vi "UHR-Fleezers Control (host) -Leonardo 04-2018 V3.vi"(0 "Tab Control":T5(tab)=enum."Trap Control (RF)") -> ()   [LabVIEW 2013] (continued)
                n951 = Unbundle By Name(w1533) -> ("Pump 2"=w1539:T33)
                n952 = call "Set pump parameters.vi"("Pump write delay (ms)"=w1534, "Volume (uL)"="Flush Center Ch Volume (uL)", "Rate (uL/h)"=w1530, "Units"=3.0, "Pump #"=2.0, "Pump Parameters In"=w1539, "VISA resource name"=w1538) -> ("Pump Parameters Out"=w1532:T33)  [unwired: 3 in]
                n953 = Bundle By Name(cluster=w1533, "Pump 2"=w1532) -> (w1531:T6)
                n954 = local write "All Pump Parameters"(w1531) -> ()
                n955 = Add(x="Flush Center Ch Volume (uL)", y="Total Volume\nFlushed (uL)") -> (x+y=w1527:dbl)
                n956 = local write "Total Volume\nFlushed (uL)"(w1527) -> ()
              }
              frame #1 {
                n957 = Wait (ms)(milliseconds to wait=w1540) -> ()  [unwired: 1 out]
              }
              frame #2 {
                n958 = call "Write to pump.vi"("string"="start", "VISA resource name"=w1541) -> ()  [unwired: 1 out]
              }
            }
            n959 = local read "Chemyx Syringe Pump Serial Port"() -> (w1524:refnum<visa-resource-name>)
          }
          frame Enabled {
            n960 = call "hamilton_controller.vi"("Open?"=w1543, "valve"=enum16{"A", "B", "C", "D", "ALL"}."B", "action"=T21."MOVE VALVE") -> ()  [unwired: 8 in, 1 out]
          }
        }
      }
      event "Inject Bottom": Value Change {
        n961 = event-data() -> ()  [unwired: 7 out]
        n962 = call "hamilton_controller.vi"("Open?"="Inject Bottom", "valve"=enum16{"A", "B", "C", "D", "ALL"}."C", "action"=T21."MOVE VALVE") -> ()  [unwired: 8 in, 1 out]
      }
      event "Shunt:": Value Change {
        n963 = event-data() -> ()  [unwired: 7 out]
        n964 = call "hamilton_controller.vi"("Open?"="Shunt:", "valve"=enum16{"A", "B", "C", "D", "ALL"}."D", "action"=T21."MOVE VALVE") -> ()  [unwired: 8 in, 1 out]
      }
      event "Flip Green Filter": Value Change {
        n965 = event-data() -> ()  [unwired: 7 out]
        n966 = local write "Flip Green Filter"("Flip Green Filter") -> ()
        n967 = flat-sequence {
          tunnel: w1559 -> [w1564]
          tunnel: w1558 -> [w1563]
          tunnel: [w1561] -> w1556
          tunnel: [w1560] -> w1555
          tunnel: [w1566] -> w1554
          tunnel: w1556 -> [w1566]
          tunnel: [w1565] -> w1553
          tunnel: w1555 -> [w1565]
          tunnel: w1554 -> [w1570]
          tunnel: w1553 -> [w1569]
          tunnel: [w1568] -> w1557
          frame #0 {
            n968 = xnode "Read/Write Control"("FPGA VI Reference In"=w1564, "error in"=w1563, "Green Filter Flipper"=TRUE) -> ("FPGA VI Reference Out"=w1561:T20, "error out"=w1560:errorcluster)
          }
          frame #1 {
            n969 = Wait (ms)(milliseconds to wait=u32 100) -> ()  [unwired: 1 out]
          }
          frame #2 {
            n970 = xnode "Read/Write Control"("FPGA VI Reference In"=w1570, "error in"=w1569, "Green Filter Flipper"=FALSE) -> ("error out"=w1568:errorcluster)  [unwired: 1 out]
          }
        }
      }
      event "Pump 1 contents", "Pump 3 contents": Value Change {
        n971 = event-data() -> ()  [unwired: 7 out]
        n972 = local read "Pump 1 contents"() -> (→"Pump 1 cont disp":string)
        n973 = local read "Pump 3 contents"() -> (→"Pump 3 cont disp":string)
      }
      event "Reset Trap Pos. FB": Value Change {
        n974 = event-data() -> ()  [unwired: 7 out]
        n975 = xnode "Read/Write Control"("FPGA VI Reference In"=w1576, "error in"=w1575, "Trap Pos. FB Reset"="Reset Trap Pos. FB") -> ()  [unwired: 2 out]
      }
      event "Trap Pos. FB ON": Value Change {
        n976 = event-data() -> ()  [unwired: 7 out]
        n977 = xnode "Read/Write Control"("FPGA VI Reference In"=w1591, "error in"=w1590) -> ("FPGA VI Reference Out"=w1588:T20, "BD1 Frequency Out 1"=w1585:u64)  [unwired: 1 out]
        n978 = To Double Precision Float(number=w1585) -> (double precision float=w1584:dbl)
        n979 = Multiply(x=49125000.0, y=6.0) -> (x*y=w1583:dbl)
        n980 = Multiply(x=w1584, y=w1583) -> (x*y=w1581:dbl)
        n981 = Scale By Power Of 2(n=-48, x=w1581) -> (x*2^n=w1580:dbl)
        n982 = Divide(x=w1580, y=1000000.0) -> (x/y=w1577:dbl)
        n983 = flat-sequence {
          tunnel: [w1594] -> w1589
          tunnel: w1588 -> [w1595]
          tunnel: w1585 -> [w1593]
          tunnel: "Trap Pos. FB ON" -> [w1592]
          tunnel: "Trap Pos. FB ON" -> [w1601]
          tunnel: w1589 -> [w1600]
          tunnel: "Trap Pos. FB ON" -> [w1603]
          tunnel: w1577 -> [w1602]
          frame #0 {
            n984 = case shown="False" w1592 {
              tunnel: w1595 -> [w1598 w1599]
              tunnel: [w1597 w1599] -> w1594
              tunnel: w1593 -> [w1596 _]
              frame False {
                n985 = xnode "Read/Write Control"("FPGA VI Reference In"=w1598, "BD 1 Frequency 1"=w1596) -> ("FPGA VI Reference Out"=w1597:T20)  [unwired: 1 in, 1 out]
              }
              frame True {
              }
            }
          }
          frame #1 {
            n986 = xnode "Read/Write Control"("FPGA VI Reference In"=w1600, "Force feedback"=w1601) -> ()  [unwired: 1 in, 2 out]
          }
          frame #2 {
            n987 = case shown="False" w1603 {
              tunnel: w1602 -> [w1605 _]
              frame False {
                n988 = Subtract(x=90.0, y=w1605) -> (x-y=w1604:dbl)
                n989 = property on="Trap Delta (MHz)" class="DigNum (strict)"("Val(Sgnl)"=w1604) -> ()  [unwired: 2 in, 2 out]
              }
              frame True {
              }
            }
          }
        }
      }
      event "Diff. FB.", "Trap Pos. FB Gains", "Trap Pos. FB Mult Factor", "Trap Pos. FB Offset Factor", "Trap Pos FB Negate Action", "Trap Pos FB Monitor\nT1 or T2", "Negate Diff?": Value Change {
        n990 = event-data() -> ()  [unwired: 7 out]
        n991 = xnode "Read/Write Control"("FPGA VI Reference In"=w1617, "error in"=w1616, "Trap pos. FB Range"="Trap Pos. FB Range", "Trap Pos. FB Gains"="Trap Pos. FB Gains", "Trap Pos. FB Mult Factor"="Trap Pos. FB Mult Factor", "Trap Pos. FB Offset Factor"="Trap Pos. FB Offset Factor", "Trap Pos FB Negate Action"="Trap Pos FB Negate Action", "Trap Pos FB Monitor T1 or T2"="Trap Pos FB Monitor\nT1 or T2", "AI1 X Scale"="Trap Pos. AI1 X Pre-scale", "Negate Diff?"="Negate Diff?", "Diff FB Measurement?"="Diff. FB.") -> ()  [unwired: 2 out]
      }
      event "Trap Pos FB SP": Value Change {
        n992 = event-data() -> ()  [unwired: 7 out]
        n993 = xnode "Read/Write Control"("FPGA VI Reference In"=w1620, "error in"=w1619, "Trap Pos. FB SP"="Trap Pos FB SP") -> ()  [unwired: 2 out]
      }
      event "Simulate stepping": Value Change {
        n994 = event-data() -> ()  [unwired: 7 out]
        n995 = flat-sequence {
          tunnel: w1622 -> [w1625]
          tunnel: [w1624] -> _
          tunnel: w1621 -> [w1623]
          frame #0 {
            n996 = while {
              tunnel: w1625 -> [w1653]
              tunnel: [w1652] -> w1624 mode=indexing
              tunnel: w1623 -> [w1651]
              i -> [w1637]
              stop <- w1634 stop-if-true
              w1627 = 1000.0
              n997 = Divide(x="Backtrack probability", y=100) -> (x/y=w1661:dbl)
              n998 = Random Number (0-1)() -> (number: 0 to 1=w1662:dbl)
              n999 = Greater?(x=w1662, y=w1661) -> (0:w1660:bool)
              n1000 = Select(t=1, s=w1660, f=-1) -> (s? t:f=w1657:i32)
              n1001 = local read "BD 1 Frequency 2 (MHz)"() -> (w1632:dbl)
              n1002 = Multiply(x=w1657, y="Step size (nm)") -> (x*y=w1655:dbl)
              "Step taken" <- w1655
              n1003 = Divide(x=w1655, y=168.33) -> (x/y=w1630:dbl)
              n1004 = local read "BD 1 Frequency 1 (MHz)"() -> (w1631:dbl)
              n1005 = local read "X RF Frequency Limits (MHz)"() -> (w1650:T16)
              n1006 = local read "Y RF Frequency Limits (MHz)"() -> (w1649:T16)
              n1007 = Subtract(x=w1631, y=w1630) -> (x-y=w1629:dbl)
              n1008 = local write "BD 1 Frequency 1 (MHz)"(w1629) -> ()
              n1009 = local read "BD 2 Frequency 1 (MHz)"() -> (w1647:dbl)
              n1010 = local read "BD 2 Frequency 2 (MHz)"() -> (w1648:dbl)
              n1011 = call "set RF board frequency - interlace.vi"("Board 2 Frequency Limits"=w1649, "Board 1 Frequency Limits"=w1650, "error in"=w1653, "FPGA VI Reference In"=w1651, "Board 2 Frequency 2 (MHz)"=w1648, "Board 2 Frequency 1 (MHz)"=w1647, "Board 1 Frequency 2 (MHz)"=w1632, "Board 1 Frequency 1  (MHz)"=w1629) -> ("error out"=w1652:errorcluster)  [unwired: 2 in, 1 out]
              n1012 = Subtract(x=w1632, y=w1629) -> (x-y=w1646:dbl)
              n1013 = Subtract(x=w1648, y=w1647) -> (x-y=w1645:dbl)
              n1014 = Square(x=w1645) -> (x^2=w1643:dbl)
              n1015 = Square(x=w1646) -> (x^2=w1644:dbl)
              n1016 = Add(x=w1644, y=w1643) -> (x+y=w1642:dbl)
              n1017 = Square Root(x=w1642) -> (sqrt(x)=w1633:dbl)
              n1018 = local write "Trap Delta (MHz)"(w1633) -> ()
              n1019 = property on="Initial delta (MHz)" class="DigNum (strict)"("Val(Sgnl)"=w1633) -> ()  [unwired: 2 in, 2 out]
              n1020 = Multiply(x="Mean dwell time (s)", y=w1627) -> (x*y=w1639:dbl)
              n1021 = case shown="\"Gamma2\"" "Distribution" {
                tunnel: w1639 -> [w1666 w1670 w1673]
                tunnel: [w1666 w1667 w1674] -> w1628
                frame "uniform", Default {
                }
                frame "Exponential" {
                  n1022 = call-poly <vilib>:"Continuous Random.vi"("b"=w1670, "samples"=1) -> ("exp random data"=w1668:dbl[])  [unwired: 8 in, 1 out]
                  n1023 = Index Array(array=w1668) -> (element=w1667:dbl)  [unwired: 1 in]
                }
                frame "Gamma2" {
                  w1671 = 2.0
                  # "Note: the shape and scale\nparameters of the gamma\nare inverted because LabView..."
                  n1024 = Divide(x=w1673, y=w1671) -> (x/y=w1672:dbl)
                  n1025 = call-poly <vilib>:"Continuous Random.vi"("c"=w1672, "b"=w1671, "samples"=1) -> ("gamma random numbers"=w1675:dbl[])  [unwired: 7 in, 1 out]
                  n1026 = Index Array(array=w1675) -> (element=w1674:dbl)  [unwired: 1 in]
                }
              }
              n1027 = Divide(x=w1628, y=w1627) -> (x/y=→"Step duration":dbl)
              n1028 = To Unsigned Long Integer(number=w1628) -> (unsigned 32bit integer=w1640:u32)
              n1029 = Add(x=w1637, y=1) -> (x+y=w1636:i32)
              n1030 = Wait (ms)(milliseconds to wait=w1640) -> ()  [unwired: 1 out]
              n1031 = Equal?(x=w1636, y="Number of steps") -> (x = y?=w1634:bool)
            }
          }
          frame #1 {
            n1032 = local write "Simulate stepping"(FALSE) -> ()
          }
        }
      }
      event "Set SP to Reading": Value Change {
        n1033 = event-data() -> ()  [unwired: 7 out]
        n1034 = local read "Trap Pos FB Monitor\nT1 or T2"() -> (w1685:bool)
        n1035 = local read "Trap X AI1 (DMA)"() -> (w1688:T13)
        n1036 = local read "Trap X (AI1)"() -> (w1691:T1)
        n1037 = Unbundle By Name(w1691) -> ("Trap 1"=w1690:fxp<+/-,16,1>, "Trap 2"=w1689:fxp<+/-,16,1>)
        n1038 = Unbundle By Name(w1688) -> ("Set 1"=w1687:fxp<+/-,16,1>, "Set 2"=w1686:fxp<+/-,16,1>)
        n1039 = Select(t=w1690, s=w1685, f=w1689) -> (s? t:f=w1684:fxp<+/-,16,1>)
        n1040 = Select(t=w1687, s=w1685, f=w1686) -> (s? t:f=w1683:fxp<+/-,16,1>)
        n1041 = Not(x="Set SP Using...") -> (.not. x?=w1678:bool)
        n1042 = Select(t=w1684, s=w1678, f=w1683) -> (s? t:f=w1679:fxp<+/-,16,1>)
        n1043 = xnode "Read/Write Control"("FPGA VI Reference In"=w1681, "error in"=w1680, "Trap Pos. FB SP"=w1679) -> ()  [unwired: 2 out]
        n1044 = local write "Trap Pos FB SP"(w1679) -> ()
      }
      event "Trap Pos. FB Out Scale 2^n": Value Change {
        n1045 = event-data() -> ()  [unwired: 7 out]
        n1046 = Scale By Power Of 2(n="Trap Pos. FB Out Scale 2^n", x=ext 1.0) -> (x*2^n=w1693:ext)
        n1047 = property on="Trap Pos. FB Mult Factor" class="DigNum (strict)"("Val(Sgnl)"=w1693) -> ()  [unwired: 2 in, 2 out]
      }
      event "Trap Pos FB Int Count": Value Change {
        n1048 = event-data() -> ()  [unwired: 7 out]
        n1049 = xnode "Read/Write Control"("FPGA VI Reference In"=w1698, "error in"=w1697, "Trap Pos FB Int Count"="Trap Pos FB Int Count") -> ()  [unwired: 2 out]
      }
      event "Target Force (pN)", "Setpoint offset\nCorrection values", "Raster target force (pN)": Value Change {
        w1706 = 2.0
        n1050 = event-data() -> ()  [unwired: 7 out]
        n1051 = local read "B factor"() -> (w1737:dbl)
        n1052 = To Fixed-Point(number=w1737) -> (fixed-point=w1736:fxp<+/-,16,16>)  [unwired: 1 in]
        n1053 = xnode "Read/Write Control"("FPGA VI Reference In"=w1700, "B factor"=w1736) -> ("BD1 Frequency Out 1"=w1727:u64)  [unwired: 1 in, 2 out]
        n1054 = local read "BD 1 Frequency 2 (MHz)"() -> (w1726:dbl)
        n1055 = local read "Target Force (pN)"() -> (w1712:dbl)
        n1056 = To Double Precision Float(number=w1727) -> (double precision float=w1733:dbl)
        n1057 = Multiply(x=49125000.0, y=6.0) -> (x*y=w1732:dbl)
        n1058 = Multiply(x=w1733, y=w1732) -> (x*y=w1730:dbl)
        n1059 = Scale By Power Of 2(n=-48, x=w1730) -> (x*2^n=w1729:dbl)
        n1060 = Divide(x=w1729, y=1000000.0) -> (x/y=w1725:dbl)
        n1061 = Subtract(x=w1726, y=w1725) -> (x-y=w1724:dbl)
        n1062 = local read "T1 kappa_x (pN/nm)"() -> (w1713:dbl)
        n1063 = local read "T1 alpha_x (nm/V)"() -> (w1714:dbl)
        n1064 = local read "Negate offset difference"() -> (w1715:bool)
        n1065 = local read "Offset file step size"() -> (w1723:dbl)
        n1066 = Multiply(x="Raster target force (pN)", y=w1706) -> (x*y=w1705:dbl)
        n1067 = Multiply(x=w1712, y=w1706) -> (x*y=w1711:dbl)
        n1068 = local read "Setpoint offset\nCorrection values"() -> (w1720:dbl[])
        n1069 = Divide(x=w1724, y=w1723) -> (x/y=w1722:dbl)
        n1070 = Select(t=-1, s=w1715, f=1) -> (s? t:f=w1716:i32)
        n1071 = To Long Integer(number=w1722) -> (32bit integer=w1721:i32)
        n1072 = Multiply(x=w1714, y=w1713) -> (x*y=w1704:dbl)
        n1073 = Divide(x=w1711, y=w1704) -> (x/y=w1710:dbl)
        n1074 = Index Array(array=w1720, index=w1721) -> (element=w1719:dbl)
        n1075 = Divide(x=w1705, y=w1704) -> (x/y=w1703:dbl)
        n1076 = Multiply(x=w1716, y=w1719) -> (x*y=w1702:dbl)
        n1077 = Add(x=w1710, y=w1702) -> (x+y=w1709:dbl)
        n1078 = Add(x=w1703, y=w1702) -> (x+y=w1701:dbl)
        n1079 = To Fixed-Point(number=w1701) -> (fixed-point=w1699:fxp<+/-,16,1>)  [unwired: 1 in]
        n1080 = To Fixed-Point(number=w1709) -> (fixed-point=w1708:fxp<+/-,16,1>)  [unwired: 1 in]
        n1081 = property on="Trap Pos FB SP" class="DigNum (strict)"("Val(Sgnl)"=w1708) -> ()  [unwired: 2 in, 2 out]
        n1082 = xnode "Read/Write Control"("FPGA VI Reference In"=w1700, "Raster setpoint"=w1699) -> ()  [unwired: 1 in, 2 out]
      }
      event "Read setpoint correction\nfile": Value Change {
        n1083 = event-data() -> ()  [unwired: 7 out]
        n1084 = local write "Read setpoint correction\nfile"(FALSE) -> ()
        n1085 = Open/Create/Replace File(file path (use dialog)="Setpoint correction\noffset file", operation (0:open)=T24."open", access (0:read/write)=enum16{"read/write", "read-only", "write-only"}."read-only") -> (refnum out=w1762:refnum<file>)  [unwired: 1 in, 4 out]
        n1086 = Deny Access(7:w1762) -> (3:w1760:refnum<file>)  [unwired: 1 in, 2 out]
        n1087 = Read from Binary File(5:0.0, 9:T30."big-endian, network order" ("byte order (0:big-endian, network order)"), 10:-1 ("count (1)"), 11:w1760) -> (2:w1753:dbl[], 3:w1759:refnum<file>)  [unwired: 1 in, 3 out]
        n1088 = Close File(refnum=w1759) -> ()  [unwired: 1 in, 2 out]
        n1089 = Index Array(array=w1753, index=0) -> (element=w1749:dbl)
        n1090 = local write "Offset file step size"(w1749) -> ()
        n1091 = Array Subset(array=w1753, index=3) -> (w1752:dbl[])  [unwired: 1 in]
        n1092 = local read "T1 kappa_x (pN/nm)"() -> (w1747:dbl)
        n1093 = local read "T1 alpha_x (nm/V)"() -> (w1748:dbl)
        n1094 = local read "T2 alpha_x (nm/V)"() -> (w1746:dbl)
        n1095 = local read "T2 kappa_x (pN/nm)"() -> (w1745:dbl)
        n1096 = Decimate 1D Array(w1752) -> (w1740:dbl[], w1741:dbl[])  [unwired: 1 out]
        n1097 = local read "Offset Values"() -> (w1751:T14)
        n1098 = Multiply(x=w1748, y=w1747) -> (x*y=w1743:dbl)
        n1099 = Multiply(x=w1746, y=w1745) -> (x*y=w1744:dbl)
        n1100 = Bundle By Name(cluster=w1751, "Trap 1X offset"=w1740, "Trap 2X offset"=w1741) -> (w1750:T14)
        n1101 = Divide(x=w1744, y=w1743) -> (x/y=w1742:dbl)
        n1102 = property on="B factor" class="DigNum (strict)"("Val(Sgnl)"=w1742) -> ()  [unwired: 2 in, 2 out]
        n1103 = Multiply(x=w1741, y=w1742) -> (x*y=w1739:dbl[])
        n1104 = local write "Offset Values"(w1750) -> ()
        n1105 = Subtract(x=w1740, y=w1739) -> (x-y=w1738:dbl[])
        n1106 = property on="Setpoint offset\nCorrection values" class="Arr (strict)"("Val(Sgnl)"=w1738) -> ()  [unwired: 2 in, 2 out]
      }
      event "MCL Tracking": Value Change {
        n1107 = event-data() -> ()  [unwired: 7 out]
        n1108 = case shown="True" "MCL Tracking" {
          frame False {
            n1109 = local read "Current MCL (V)"() -> (w1767:dbl)
            n1110 = local write "AO2"(w1767) -> ()
          }
          frame True {
            n1111 = local read "BD 1 Frequency 1 (MHz)"() -> (→"Zero T1 position":dbl)
            n1112 = local read "AO2"() -> (→"Zero MCL x position":dbl)
          }
        }
      }
      event "Long - scale interlacing", "Cycles ON", "Cycles OFF": Value Change {
        n1113 = event-data() -> ()  [unwired: 7 out]
        n1114 = local read "Long - scale interlacing"() -> (w1772:bool)
        n1115 = local read "Cycles OFF"() -> (w1770:i16)
        n1116 = local read "Cycles ON"() -> (w1771:i16)
        n1117 = xnode "Read/Write Control"("FPGA VI Reference In"=w1773, "Number of OFF cycles"=w1770, "Number of ON cycles"=w1771, "Green long-scale interlacing"=w1772) -> ()  [unwired: 1 in, 2 out]
      }
      event "Scale intensities": Value Change {
        n1118 = event-data() -> ()  [unwired: 7 out]
        n1119 = local read "Trap Intensity\nSetpoints (V)"() -> (w1777:cluster{"Set 1":dbl, "Set 2":dbl})
        n1120 = local read "T1 kappa_x (pN/nm)"() -> (w1783:dbl)
        n1121 = local read "T2 kappa_x (pN/nm)"() -> (w1782:dbl)
        n1122 = Unbundle By Name(w1777) -> ("Set 1"=w1779:dbl, "Set 2"=w1778:dbl)
        n1123 = case shown="False" "Scale intensities" {
          tunnel: "Scale factor" -> [w1793 w1805]
          tunnel: "Scale factor" -> [w1788 w1798]
          tunnel: w1783 -> [w1795 w1804]
          tunnel: w1782 -> [w1794 w1803]
          tunnel: [w1791 w1802] -> w1781
          tunnel: [w1792 w1801] -> w1780
          tunnel: w1779 -> [w1790 w1800]
          tunnel: w1778 -> [w1789 w1799]
          tunnel: [w1787 w1797] -> w1776
          tunnel: [w1786 w1796] -> w1775
          frame False {
            n1124 = Divide(x=w1795, y=w1788) -> (x/y=w1791:dbl)
            n1125 = Divide(x=w1794, y=w1793) -> (x/y=w1792:dbl)
            n1126 = Divide(x=w1790, y=w1788) -> (x/y=w1787:dbl)
            n1127 = Divide(x=w1789, y=w1788) -> (x/y=w1786:dbl)
          }
          frame True {
            n1128 = Multiply(x=w1800, y=w1798) -> (x*y=w1797:dbl)
            n1129 = Multiply(x=w1799, y=w1798) -> (x*y=w1796:dbl)
            n1130 = Multiply(x=w1804, y=w1798) -> (x*y=w1802:dbl)
            n1131 = Multiply(x=w1805, y=w1803) -> (x*y=w1801:dbl)
          }
        }
        n1132 = local write "T2 kappa_x (pN/nm)"(w1780) -> ()
        n1133 = local write "T1 kappa_x (pN/nm)"(w1781) -> ()
        n1134 = Bundle By Name(cluster=w1777, "Set 1"=w1776, "Set 2"=w1775) -> (w1774:cluster{"Set 1":dbl, "Set 2":dbl})
        n1135 = local write "Trap Intensity\nSetpoints (V)"(w1774) -> ()
      }
    }
    "error out 2" <- w770
    n1136 = node-c288() -> ()  [unwired: 1 in, 1 out]
  }
  n1137 = node-c288() -> (w102:T25)  [unwired: 4 in]
  n1138 = timed-loop "Run Scripts, including: stage motion" {
    timing: w102 -> [_]
    timing-out: [_] -> w101
    tunnel: w57 -> [_]
    stop <- w1807 stop-if-true
    n1139 = node-c288() -> ()  [unwired: 1 in, 1 out]
    n1140 = event shown="[5] \"Profile\": Value Change" {
      selector: _ -> [_ _ _ _ _ _ _ _ _ _ _ _]
      dyn-events: _ -> [_ _ _ _ _ _ _ _ _ _ _ _]
      timeout: 50 -> [_ _ _ _ _ _ _ _ _ _ _ _]
      tunnel: ["Move Cap. 1 (DNA Top)" _ "Cal/Data Acq. Spot" "Dump Beads" "Dip for Protein" _ "Got ADig bead" "Got DNA bead" "Take Stepping Data" _ "Take Detection Laser\nImage" _] -> _
      tunnel: [_ _ _ _ _ _ _ _ _ _ _ w2015] -> w1807
      event "Move Cap. 1 (DNA Top)": Value Change {
        n1141 = event-data() -> ()  [unwired: 1 in, 5 out]
        n1142 = local write "Move Cap. 1 (DNA Top)"(FALSE ("Move Cap. 1 (DNA Right)")) -> ()
        n1143 = flat-sequence {
          tunnel: "Cap 1 Samp Flow ON" -> [w1813]
          frame #0 {
            n1144 = local write "Stage Moving"(FALSE ("Stage Moving")) -> ()
            n1145 = case "stop flow" shown="True" w1813 {
              frame False {
              }
              frame True {
                n1146 = call "hamilton_controller.vi"("Open?"=FALSE, "valve"=enum16{"A", "B", "C", "D", "ALL"}."C", "action"=T21."MOVE VALVE") -> ()  [unwired: 8 in, 1 out]
              }
            }
            n1147 = case shown="True" TRUE {
              tunnel: "Cap 1 T ON" -> [w1822 w1823]
              frame False {
                n1148 = property on="Trap 1 (ON/OFF)" class="Bool (strict)"("Val(Sgnl)"=w1822) -> ()  [unwired: 2 in, 2 out]
              }
              frame True {
                n1149 = property on="Trap 2 (ON/OFF)" class="Bool (strict)"("Val(Sgnl)"=w1823) -> ()  [unwired: 2 in, 2 out]
              }
            }
            n1150 = call <vilib>:"Beep.vi"() -> ()  [unwired: 3 in, 9 out]
            n1151 = case shown="True" "Cap 1 Flow ON" {
              frame False {
              }
              frame True {
                n1152 = property on="Main:" class="Bool (strict)"("Val(Sgnl)"=TRUE ("Value (Signaling)")) -> ()  [unwired: 2 in, 2 out]
              }
            }
          }
        }
      }
      event Timeout {
        n1153 = event-data() -> ()  [unwired: 1 in, 2 out]
      }
      event "Cal/Data Acq. Spot": Value Change {
        # "wait for calibration file\nto be written"
        # "signal save cal true\nthis tells the data \nacquisition loop to\nstart sending the data\nto a calibration file"
        # "separate traps to\nthe desired trap delta"
        # "move stage to data acquisition spot"
        # "CHANGE FISH FOR TETHER BACK\nTO TRUE VALUE HERE."
        n1154 = event-data() -> ()  [unwired: 1 in, 5 out]
        n1155 = local write "Cal/Data Acq. Spot"(FALSE ("Cal/Data Acq. Spot")) -> ()
        n1156 = flat-sequence {
          tunnel: ["Cal @ (MHz)"] -> w1824
          tunnel: w1824 -> [w1834]
          tunnel: w1824 -> [w1855]
          frame #0 {
            n1157 = property on="Trap Delta (MHz)" class="DigNum (strict)"("Val(Sgnl)"="Cal @ (MHz)") -> ()  [unwired: 2 in, 2 out]
            n1158 = call <vilib>:"Beep.vi"() -> ()  [unwired: 3 in, 9 out]
          }
          frame #1 {
            n1159 = Wait (ms)(milliseconds to wait=u32 100) -> ()  [unwired: 1 out]
          }
          frame #2 {
            n1160 = property on="Save Calibration" class="Bool (strict)"("Val(Sgnl)"=TRUE ("Value (Signaling)")) -> ()  [unwired: 2 in, 2 out]
          }
          frame #3 {
            n1161 = Wait (ms)(milliseconds to wait=u32 4000) -> ()  [unwired: 1 out]
          }
          frame #4 {
            n1162 = while {
              stop <- w1831 stop-if-true
              n1163 = local read "Saving..."() -> (w1832:bool)
              n1164 = Wait (ms)(milliseconds to wait=u32 100) -> ()  [unwired: 1 out]
              n1165 = Not(x=w1832) -> (.not. x?=w1831:bool)
            }
          }
          frame #5 {
            n1166 = case shown="True" "W/ Offset 1" {
              tunnel: w1834 -> [_ w1836]
              frame False {
              }
              frame True {
                n1167 = stacked-sequence {
                  tunnel: w1836 -> [_ _ _ _ _ _ _ w1853]
                  frame #0 {
                    n1168 = Replace Array Subset(array=u32[] [0] ("Index Values"), new element="Offset 1 Set", index=0) -> (w1837:u32[])
                    n1169 = property on="Saved AOD Raster Scan Parameter Sets" class="Arr (strict)"("Index Values"=w1837) -> ()  [unwired: 2 in, 2 out]
                    n1170 = property on="Trap Delta (MHz)" class="DigNum (strict)"("Val(Sgnl)"="Offset 1 Start (MHz)") -> ()  [unwired: 2 in, 2 out]
                  }
                  frame #1 {
                    n1171 = Wait (ms)(milliseconds to wait=u32 200) -> ()  [unwired: 1 out]
                  }
                  frame #2 {
                    n1172 = property on="Load parameters" class="Bool (strict)"("Val(Sgnl)"=TRUE ("Value (Signaling)")) -> ()  [unwired: 2 in, 2 out]
                  }
                  frame #3 {
                    n1173 = Wait (ms)(milliseconds to wait=u32 200) -> ()  [unwired: 1 out]
                  }
                  frame #4 {
                    n1174 = property on="Trap Raster Scan" class="Bool (strict)"("Val(Sgnl)"=TRUE ("Value (Signaling)")) -> ()  [unwired: 2 in, 2 out]
                  }
                  frame #5 {
                    n1175 = Wait (ms)(milliseconds to wait=u32 2000) -> ()  [unwired: 1 out]
                  }
                  frame #6 {
                    n1176 = while {
                      stop <- w1850 stop-if-true
                      n1177 = local read "Raster Scanning..."() -> (w1852:bool)
                      n1178 = local read "Saving..."() -> (w1848:bool)
                      n1179 = Wait (ms)(milliseconds to wait=u32 100) -> ()  [unwired: 1 out]
                      n1180 = Not(x=w1848) -> (.not. x?=w1847:bool)
                      n1181 = Not(x=w1852) -> (.not. x?=w1849:bool)
                      n1182 = And(x=w1849, y=w1847) -> (x .and. y?=w1850:bool)
                    }
                  }
                  frame #7 {
                    n1183 = property on="Trap Delta (MHz)" class="DigNum (strict)"("Val(Sgnl)"=w1853) -> ()  [unwired: 2 in, 2 out]
                  }
                }
              }
            }
          }
          frame #6 {
            n1184 = local read "Save ave N"() -> (w1854:dbl)
            n1185 = case shown="True" "W/ Offset 2" {
              tunnel: w1855 -> [_ w1861]
              tunnel: w1854 -> [_ w1860]
              frame False {
                n1186 = Multiply(x="Cal read wait (s)", y=u32 1000 ("milliseconds to wait")) -> (x*y=w1858:u32)
                n1187 = Wait (ms)(milliseconds to wait=w1858) -> ()  [unwired: 1 out]
              }
              frame True {
                n1188 = stacked-sequence {
                  tunnel: w1861 -> [_ _ _ _ _ _ _ _ _ w1882 _ _]
                  tunnel: w1860 -> [_ _ _ _ _ _ _ _ _ w1880 _ _]
                  frame #0 {
                    n1189 = property on="Save ave N" class="DigNum (strict)"("Val(Sgnl)"=1.0 ("Value (Signaling)")) -> ()  [unwired: 2 in, 2 out]
                  }
                  frame #1 {
                    n1190 = Wait (ms)(milliseconds to wait=u32 500) -> ()  [unwired: 1 out]
                  }
                  frame #2 {
                    n1191 = property on="Trap Delta (MHz)" class="DigNum (strict)"("Val(Sgnl)"="Offset 2 Start (MHz)") -> ()  [unwired: 2 in, 2 out]
                    n1192 = Replace Array Subset(array=u32[] [0] ("Index Values"), new element="Offset 2 Set", index=0) -> (w1866:u32[])
                    n1193 = property on="Saved AOD Raster Scan Parameter Sets" class="Arr (strict)"("Index Values"=w1866) -> ()  [unwired: 2 in, 2 out]
                  }
                  frame #3 {
                    n1194 = Wait (ms)(milliseconds to wait=u32 500) -> ()  [unwired: 1 out]
                  }
                  frame #4 {
                    n1195 = property on="Load parameters" class="Bool (strict)"("Val(Sgnl)"=TRUE ("Value (Signaling)")) -> ()  [unwired: 2 in, 2 out]
                  }
                  frame #5 {
                    n1196 = Wait (ms)(milliseconds to wait=u32 500) -> ()  [unwired: 1 out]
                  }
                  frame #6 {
                    n1197 = property on="Trap Raster Scan" class="Bool (strict)"("Val(Sgnl)"=TRUE ("Value (Signaling)")) -> ()  [unwired: 2 in, 2 out]
                  }
                  frame #7 {
                    n1198 = Wait (ms)(milliseconds to wait=u32 2000) -> ()  [unwired: 1 out]
                  }
                  frame #8 {
                    n1199 = while {
                      stop <- w1875 stop-if-true
                      n1200 = local read "Raster Scanning..."() -> (w1878:bool)
                      n1201 = local read "Saving..."() -> (w1876:bool)
                      n1202 = Wait (ms)(milliseconds to wait=u32 100) -> ()  [unwired: 1 out]
                      n1203 = Not(x=w1876) -> (.not. x?=w1874:bool)
                      n1204 = Not(x=w1878) -> (.not. x?=w1877:bool)
                      n1205 = And(x=w1877, y=w1874) -> (x .and. y?=w1875:bool)
                    }
                  }
                  frame #9 {
                    n1206 = property on="Trap Delta (MHz)" class="DigNum (strict)"("Val(Sgnl)"=w1882) -> ()  [unwired: 2 in, 2 out]
                    n1207 = property on="Saved AOD Raster Scan Parameter Sets" class="Arr (strict)"("Index Values"=u32[] [0]) -> ()  [unwired: 2 in, 2 out]
                    n1208 = property on="Save ave N" class="DigNum (strict)"("Val(Sgnl)"=w1880) -> ()  [unwired: 2 in, 2 out]
                  }
                  frame #10 {
                    n1209 = Wait (ms)(milliseconds to wait=u32 500) -> ()  [unwired: 1 out]
                  }
                  frame #11 {
                    n1210 = property on="Load parameters" class="Bool (strict)"("Val(Sgnl)"=TRUE ("Value (Signaling)")) -> ()  [unwired: 2 in, 2 out]
                  }
                }
              }
            }
          }
          frame #7 {
            n1211 = property on="Read Cal" class="Bool (strict)"("Val(Sgnl)"=TRUE ("Value (Signaling)")) -> ()  [unwired: 2 in, 2 out]
          }
          frame #8 {
            n1212 = Wait (ms)(milliseconds to wait=u32 500) -> ()  [unwired: 1 out]
          }
          frame #9 {
            n1213 = property on="Fish for Tether" class="Bool (strict)"("Val(Sgnl)"=FALSE ("Value (Signaling)")) -> ()  [unwired: 2 in, 2 out]
          }
        }
      }
      event "Dump Beads": Value Change {
        # "SCRIPT TO REMOVE BOTH BEADS FROM THE TRAPS. TURNS ON LIGHT WHICH INDICATES THAT STAGE IS MOVING. THEN STOPS SAVING DATA. \nSETS Sample Channel Flow TO TRUE. STOPS INTERLACING GREEN FLUORESCENCE. TURNS OFF Tether INDICATOR BECAUSE WE ARE THROWING IT\nAWAY. SHUTS OFF TRAP POSITION FEEDBACK."
        n1214 = event-data() -> ()  [unwired: 1 in, 5 out]
        n1215 = flat-sequence {
          frame #0 {
            w1889 = FALSE ("Fl. Triggered...")
            w1890 = TRUE ("Stage Moving")
            n1216 = local read "Saving..."() -> (w1891:bool)
            n1217 = local write "Fl. Triggered..."(w1889) -> ()
            n1218 = local write "Stage Moving"(w1890) -> ()
            n1219 = local write "Tether"(w1889) -> ()
            n1220 = property on="Green Laser ON/Interlacing" class="Bool (strict)"("Val(Sgnl)"=w1889) -> ()  [unwired: 2 in, 2 out]
            n1221 = property on="Trap Pos. FB ON" class="Bool (strict)"("Val(Sgnl)"=w1889) -> ()  [unwired: 2 in, 2 out]
            n1222 = property on="Inject Bottom" class="Bool (strict)"("Val(Sgnl)"=w1890) -> ()  [unwired: 2 in, 2 out]
            n1223 = local write "Stop Saving"(w1891) -> ()
          }
          frame #1 {
            w1892 = FALSE ("Value (Signaling)")
            # "TURNS TRAPS OFF SO THAT\nBEADS REMAIN AT DUMP \nBEADS POSITION"
            n1224 = property on="Trap 1 (ON/OFF)" class="Bool (strict)"("Val(Sgnl)"=w1892) -> ()  [unwired: 2 in, 2 out]
            n1225 = property on="Trap 2 (ON/OFF)" class="Bool (strict)"("Val(Sgnl)"=w1892) -> ()  [unwired: 2 in, 2 out]
            n1226 = call <vilib>:"Beep.vi"() -> ()  [unwired: 3 in, 9 out]
          }
          frame #2 {
            n1227 = property on="Goto Bottom (F7)" class="Bool (strict)"("Val(Sgnl)"=TRUE ("Value (Signaling)")) -> ()  [unwired: 2 in, 2 out]
          }
          frame #3 {
            n1228 = Wait (ms)(milliseconds to wait=u32 8000) -> ()  [unwired: 1 out]
          }
          frame #4 {
            n1229 = property on="Trap Delta (MHz)" class="DigNum (strict)"("Val(Sgnl)"=20.0 ("Value (Signaling)")) -> ()  [unwired: 2 in, 2 out]
          }
          frame #5 {
            n1230 = property on="Trap 2 (ON/OFF)" class="Bool (strict)"("Val(Sgnl)"=TRUE ("Value (Signaling)")) -> ()  [unwired: 2 in, 2 out]
          }
          frame #6 {
            n1231 = property on="Inject Bottom" class="Bool (strict)"("Val(Sgnl)"=FALSE ("Value (Signaling)")) -> ()  [unwired: 2 in, 2 out]
          }
        }
      }
      event "Dip for Protein": Value Change {
        n1232 = event-data() -> ()  [unwired: 1 in, 5 out]
        n1233 = flat-sequence {
          frame #0 {
            n1234 = case shown="True" "Move Trap Before?" {
              frame False {
              }
              frame True {
                n1235 = property on="Trap Delta (MHz)" class="DigNum (strict)"("Val(Sgnl)"="Dip Trap Delta 1 (MHz)") -> ()  [unwired: 2 in, 2 out]
              }
            }
          }
          frame #1 {
            n1236 = Multiply(x="Duration (s)", y=1000.0) -> (x*y=w1901:dbl)
            n1237 = Wait (ms)(milliseconds to wait=w1901) -> ()  [unwired: 1 out]
          }
          frame #2 {
            n1238 = case shown="True" "Move Trap After?" {
              frame False {
              }
              frame True {
                n1239 = property on="Trap Delta (MHz)" class="DigNum (strict)"("Val(Sgnl)"="Dip Trap Delta 2 (MHz)") -> ()  [unwired: 2 in, 2 out]
              }
            }
          }
          frame #3 {
            n1240 = case shown="True" "Green ON After?" {
              frame False {
              }
              frame True {
                n1241 = property on="Green Laser ON/Interlacing" class="Bool (strict)"("Val(Sgnl)"=TRUE ("Value (Signaling)")) -> ()  [unwired: 2 in, 2 out]
              }
            }
          }
          frame #4 {
            n1242 = Wait (ms)(milliseconds to wait=u32 500) -> ()  [unwired: 1 out]
          }
          frame #5 {
            n1243 = case shown="True" "Save Data After?" {
              frame False {
              }
              frame True {
                n1244 = property on="Start Saving" class="Bool (strict)"("Val(Sgnl)"=TRUE ("Value (Signaling)")) -> ()  [unwired: 2 in, 2 out]
              }
            }
          }
        }
      }
      event "Profile": Value Change {
        n1245 = event-data() -> ()  [unwired: 1 in, 5 out]
        n1246 = flat-sequence {
          frame #0 {
            w1911 = 0.0 ("element")
            n1247 = Build Array(w1911, "Y change (mm)", w1911) -> ()  [unwired: 1 out]
          }
          frame #1 {
            # "stop saving"
            n1248 = local write "Stop Saving"(TRUE ("Stop Saving")) -> ()
            n1249 = local write "Stage Moving"(FALSE ("Stage Moving")) -> ()
          }
        }
      }
      event "Got ADig bead": Value Change {
        n1250 = event-data() -> ()  [unwired: 1 in, 5 out]
        n1251 = property on="Move Cap. 1 (DNA Top)" class="Bool (strict)"("Val(Sgnl)"=TRUE ("Value (Signaling)")) -> ()  [unwired: 2 in, 2 out]
        n1252 = property on="Inject Top:" class="Bool (strict)"("Val(Sgnl)"=FALSE ("Value (Signaling)")) -> ()  [unwired: 2 in, 2 out]
      }
      event "Got DNA bead": Value Change {
        n1253 = event-data() -> ()  [unwired: 1 in, 5 out]
        n1254 = property on="Cal/Data Acq. Spot" class="Bool (strict)"("Val(Sgnl)"=TRUE ("Value (Signaling)")) -> ()  [unwired: 2 in, 2 out]
        n1255 = property on="Main:" class="Bool (strict)"("Val(Sgnl)"=FALSE ("Value (Signaling)")) -> ()  [unwired: 2 in, 2 out]
      }
      event "Take Stepping Data": Value Change {
        n1256 = event-data() -> ()  [unwired: 1 in, 5 out]
        n1257 = local read "Save ave N"() -> (w1929:dbl)
        n1258 = flat-sequence {
          tunnel: w1929 -> [w1931]
          tunnel: [w1931] -> w1924
          tunnel: [w1933] -> w1925
          tunnel: w1924 -> [w1933]
          tunnel: [w1935] -> w1926
          tunnel: w1925 -> [w1935]
          tunnel: [w1938] -> w1927
          tunnel: w1926 -> [w1938]
          tunnel: [w1940] -> w1928
          tunnel: w1927 -> [w1940]
          tunnel: [w1942] -> w1922
          tunnel: w1928 -> [w1942]
          tunnel: w1922 -> [w1945]
          tunnel: [w1945] -> w1921
          tunnel: w1921 -> [w1946]
          tunnel: [w1946] -> w1923
          tunnel: w1923 -> [w1952]
          frame #0 {
            n1259 = property on="Save ave N" class="DigNum (strict)"("Val(Sgnl)"="Save ave factor") -> ()  [unwired: 2 in, 2 out]
          }
          frame #1 {
            n1260 = Wait (ms)(milliseconds to wait=u32 100) -> ()  [unwired: 1 out]
          }
          frame #2 {
            n1261 = local read "Offset 2 Start (MHz)"() -> (w1937:dbl)
            n1262 = property on="Saved AOD Raster Scan Parameter Sets" class="Arr (strict)"("Index Values"=u32[] [2]) -> ()  [unwired: 2 in, 2 out]
            n1263 = property on="Trap Delta (MHz)" class="DigNum (strict)"("Val(Sgnl)"=w1937) -> ()  [unwired: 2 in, 2 out]
          }
          frame #3 {
            n1264 = property on="Load parameters" class="Bool (strict)"("Val(Sgnl)"=TRUE ("Value (Signaling)")) -> ()  [unwired: 2 in, 2 out]
          }
          frame #4 {
            n1265 = Wait (ms)(milliseconds to wait=u32 100) -> ()  [unwired: 1 out]
          }
          frame #5 {
            n1266 = property on="Trap Raster Scan" class="Bool (strict)"("Val(Sgnl)"=TRUE ("Value (Signaling)")) -> ()  [unwired: 2 in, 2 out]
          }
          frame #6 {
            n1267 = Wait (ms)(milliseconds to wait=u32 1000) -> ()  [unwired: 1 out]
          }
          frame #7 {
            n1268 = while {
              stop <- w1949 stop-if-true
              n1269 = local read "Raster Scanning..."() -> (w1951:bool)
              n1270 = local read "Saving..."() -> (w1950:bool)
              n1271 = Not(x=w1950) -> (.not. x?=w1947:bool)
              n1272 = Not(x=w1951) -> (.not. x?=w1948:bool)
              n1273 = And(x=w1948, y=w1947) -> (x .and. y?=w1949:bool)
            }
          }
          frame #8 {
            n1274 = property on="Save ave N" class="DigNum (strict)"("Val(Sgnl)"=w1952) -> ()  [unwired: 2 in, 2 out]
          }
        }
      }
      event "Step Size (nm)": Value Change {
        n1275 = event-data() -> ()  [unwired: 1 in, 5 out]
        n1276 = flat-sequence {
          frame #0 {
            n1277 = property on="Saved AOD Raster Scan Parameter Sets" class="Arr (strict)"("Index Values"=u32[] [1]) -> ()  [unwired: 2 in, 2 out]
          }
          frame #1 {
            n1278 = Multiply(x="N Steps", y="Step Size (nm)") -> (x*y=w1954:dbl)
            n1279 = property on="Scan Speed AOD (nm/s) 2" class="DigNum (strict)"("Value"="Step Size (nm)") -> ()  [unwired: 2 in, 2 out]
            n1280 = property on="Step Size AOD (nm) 2" class="DigNum (strict)"("Value"="Step Size (nm)") -> ()  [unwired: 2 in, 2 out]
            n1281 = property on="Scan Range AOD (nm) 2" class="DigNum (strict)"("Value"=w1954) -> ()  [unwired: 2 in, 2 out]
          }
        }
      }
      event "Take Detection Laser\nImage": Value Change {
        n1282 = event-data() -> ()  [unwired: 1 in, 5 out]
        n1283 = flat-sequence {
          tunnel: [w1982] -> w1972
          tunnel: [w1981] -> w1965
          tunnel: [w1980] -> w1957
          tunnel: [w1985] -> w1973
          tunnel: w1972 -> [w1985]
          tunnel: [w1984] -> w1966
          tunnel: w1965 -> [w1984]
          tunnel: [w1983] -> w1958
          tunnel: w1957 -> [w1983]
          tunnel: [w1989] -> w1974
          tunnel: w1973 -> [w1989]
          tunnel: [w1988] -> w1967
          tunnel: w1966 -> [w1988]
          tunnel: [w1987] -> w1959
          tunnel: w1958 -> [w1987]
          tunnel: [w1995] -> w1975
          tunnel: w1974 -> [w1995]
          tunnel: [w1994] -> w1968
          tunnel: w1967 -> [w1994]
          tunnel: [w1993] -> w1960
          tunnel: w1959 -> [w1993]
          tunnel: [w1999] -> w1976
          tunnel: w1975 -> [w1999]
          tunnel: [w1998] -> w1969
          tunnel: w1968 -> [w1998]
          tunnel: [w1997] -> w1961
          tunnel: w1960 -> [w1997]
          tunnel: [w2003] -> w1977
          tunnel: w1976 -> [w2003]
          tunnel: [w2002] -> w1970
          tunnel: w1969 -> [w2002]
          tunnel: [w2001] -> w1962
          tunnel: w1961 -> [w2001]
          tunnel: [w2007] -> w1978
          tunnel: w1977 -> [w2007]
          tunnel: [w2006] -> w1971
          tunnel: w1970 -> [w2006]
          tunnel: [w2005] -> w1963
          tunnel: w1962 -> [w2005]
          tunnel: w1978 -> [w2013]
          tunnel: w1971 -> [w2012]
          tunnel: [w2010] -> w1964
          tunnel: w1963 -> [w2010]
          tunnel: w1964 -> [w2014]
          frame #0 {
            n1284 = local read "Green Laser ON/Interlacing"() -> (w1982:bool)
            n1285 = local read "Green laser mode"() -> (w1981:enum32{"Laser ON", "Laser OFF", "Interlace"})
            n1286 = local read "Green FB On/Off"() -> (w1980:bool)
          }
          frame #1 {
            n1287 = property on="Green FB On/Off" class="Bool (strict)"("Val(Sgnl)"=FALSE ("Value (Signaling)")) -> ()  [unwired: 2 in, 2 out]
          }
          frame #2 {
            n1288 = property on="Green Laser ON/Interlacing" class="Bool (strict)"("Val(Sgnl)"=TRUE ("Value (Signaling)")) -> ()  [unwired: 2 in, 2 out]
            n1289 = property on="Flip Green Filter" class="Bool (strict)"("Val(Sgnl)"=TRUE ("Value (Signaling)")) -> ()  [unwired: 2 in, 2 out]
            n1290 = property on="Green laser mode" class="RadioBtnsControl (strict)"("Val(Sgnl)"=enum32{"Laser ON", "Laser OFF", "Interlace"}."Laser ON" ("Value (Signaling)")) -> ()  [unwired: 2 in, 2 out]
          }
          frame #3 {
            n1291 = Wait (ms)(milliseconds to wait=u32 500) -> ()  [unwired: 1 out]
          }
          frame #4 {
            n1292 = property on="Confocal Image" class="Bool (strict)"("Val(Sgnl)"=TRUE ("Value (Signaling)")) -> ()  [unwired: 2 in, 2 out]
          }
          frame #5 {
            n1293 = Wait (ms)(milliseconds to wait=u32 2000) -> ()  [unwired: 1 out]
          }
          frame #6 {
            n1294 = while {
              stop <- w2008 stop-if-true
              n1295 = local read "Saving..."() -> (w2009:bool)
              n1296 = Not(x=w2009) -> (.not. x?=w2008:bool)
            }
          }
          frame #7 {
            n1297 = property on="Flip Green Filter" class="Bool (strict)"("Val(Sgnl)"=TRUE ("Value (Signaling)")) -> ()  [unwired: 2 in, 2 out]
            n1298 = property on="Green Laser ON/Interlacing" class="Bool (strict)"("Val(Sgnl)"=w2013) -> ()  [unwired: 2 in, 2 out]
            n1299 = property on="Green laser mode" class="RadioBtnsControl (strict)"("Val(Sgnl)"=w2012) -> ()  [unwired: 2 in, 2 out]
          }
          frame #8 {
            n1300 = property on="Green FB On/Off" class="Bool (strict)"("Val(Sgnl)"=w2014) -> ()  [unwired: 2 in, 2 out]
          }
        }
      }
      event "Stop All": Value Change {
        n1301 = event-data() -> ()  [unwired: 1 in, 5 out]
        n1302 = local read "Stop All"() -> (w2015:bool)
      }
    }
    n1303 = node-c288() -> ()  [unwired: 1 in, 1 out]
  }
  n1304 = node-c288() -> (w109:T25)  [unwired: 4 out]
  n1305 = timed-loop "Mouse control: trap position (AOM deflection), set confocal spot from image" {
    tunnel: [w2017] -> w67
    tunnel: w57 -> [w2016]
    timing: w109 -> [_]
    timing-out: [_] -> w108
    stop <- w2017 stop-if-true
    n1306 = node-c288() -> ()  [unwired: 2 out]
    n1307 = event shown="[0] \"Pane\": Mouse Down" {
      selector: _ -> [_ _]
      dyn-events: _ -> [_ _]
      timeout: _ -> [_ _]
      tunnel: w2016 -> [w2020 _]
      event Mouse Down {
        n1308 = event-data() -> ("Time"=w2022:u32, "Coords"=w2021:T8, "Button"=w2023:u16)  [unwired: 6 out]
        n1309 = case shown="1" w2023 {
          tunnel: w2022 -> [_ _ w2126]
          tunnel: w2021 -> [_ w2060 w2124]
          tunnel: w2020 -> [_ _ w2122]
          frame 0, Default {
          }
          frame 1 {
            n1310 = property on="APD 2" class="ImageControl"() -> ("Displayed Image Position"=w2030:cluster{"Left":i32, "Top":i32})  [unwired: 2 in, 2 out]
            n1311 = property on="APD 1" class="ImageControl"() -> ("Displayed Image Position"=w2059:cluster{"Left":i32, "Top":i32})  [unwired: 2 in, 2 out]
            n1312 = property on="Detection Laser X" class="ImageControl"() -> ("Displayed Image Position"=w2056:cluster{"Left":i32, "Top":i32})  [unwired: 2 in, 2 out]
            n1313 = property on="Detection Laser Y" class="ImageControl"() -> ("Displayed Image Position"=w2055:cluster{"Left":i32, "Top":i32})  [unwired: 2 in, 2 out]
            n1314 = property on="APD 2" class="ImageControl"() -> ("Displayed Image Size"=w2029:cluster{"Width":u32, "Height":u32})  [unwired: 2 in, 2 out]
            n1315 = property on="APD 1" class="ImageControl"() -> ("Displayed Image Size"=w2057:cluster{"Width":u32, "Height":u32})  [unwired: 2 in, 2 out]
            n1316 = property on="Detection Laser X" class="ImageControl"() -> ("Displayed Image Size"=w2058:cluster{"Width":u32, "Height":u32})  [unwired: 2 in, 2 out]
            n1317 = property on="Detection Laser Y" class="ImageControl"() -> ("Displayed Image Size"=w2054:cluster{"Width":u32, "Height":u32})  [unwired: 2 in, 2 out]
            n1318 = Unbundle By Name(w2029) -> ("Width"=w2026:u32, "Height"=w2025:u32)
            n1319 = Unbundle By Name(w2030) -> ("Left"=w2028:i32, "Top"=w2027:i32)
            n1320 = Unbundle By Name(w2057) -> ("Width"=w2051:u32, "Height"=w2050:u32)
            n1321 = Unbundle By Name(w2058) -> ("Width"=w2047:u32, "Height"=w2046:u32)
            n1322 = Unbundle By Name(w2054) -> ("Width"=w2043:u32, "Height"=w2042:u32)
            n1323 = Unbundle By Name(w2059) -> ("Left"=w2053:i32, "Top"=w2052:i32)
            n1324 = Unbundle By Name(w2056) -> ("Left"=w2049:i32, "Top"=w2048:i32)
            n1325 = Unbundle By Name(w2055) -> ("Left"=w2045:i32, "Top"=w2044:i32)
            n1326 = Bundle("Left"=w2028, "Top"=w2027, "Width"=w2026, "Height"=w2025) -> (w2024:T34)  [unwired: 1 in]
            n1327 = Bundle("Left"=w2053, "Top"=w2052, "Width"=w2051, "Height"=w2050) -> (w2041:T34)  [unwired: 1 in]
            n1328 = Bundle("Left"=w2049, "Top"=w2048, "Width"=w2047, "Height"=w2046) -> (w2040:T34)  [unwired: 1 in]
            n1329 = Bundle("Left"=w2045, "Top"=w2044, "Width"=w2043, "Height"=w2042) -> (w2039:T34)  [unwired: 1 in]
            n1330 = Build Cluster Array(w2024, w2041, w2040, w2039) -> (w2038:T35)
            n1331 = for {
              tunnel: w2060 -> [w2071]
              tunnel: w2038 -> [w2072] mode=indexing
              shift-right: [w2069] -> w2036
              shift-left: TRUE -> [w2070]
              shift-right: [w2068] -> w2034
              shift-left: _ -> [w2064]
              shift-right: [w2067] -> w2033
              shift-left: _ -> [w2063]
              shift-right: [w2066] -> w2032
              shift-left: _ -> [w2062]
              shift-right: [w2065] -> w2031
              shift-left: _ -> [w2061]
              n1332 = case shown="True" w2070 {
                selector: w2070 -> [w2077 _]
                tunnel: w2072 -> [_ w2086]
                tunnel: w2071 -> [_ w2084]
                tunnel: [w2077 w2082] -> w2069
                tunnel: [w2076 w2081] -> w2068
                tunnel: [w2075 w2080] -> w2067
                tunnel: [w2074 w2079] -> w2066
                tunnel: [w2073 w2078] -> w2065
                tunnel: w2064 -> [w2076 _]
                tunnel: w2063 -> [w2075 _]
                tunnel: w2062 -> [w2074 _]
                tunnel: w2061 -> [w2073 _]
                frame False {
                }
                frame True {
                  n1333 = Unbundle(w2086) -> (w2085:T34)
                  n1334 = call "isclickinwindow.vi"("Image Param"=w2085, "Point32"=w2084) -> ("4 Y"=w2078:i32, "3 Height"=w2079:i32, "2 X"=w2080:i32, "1 Width"=w2081:i32, "In image?"=w2083:bool)  [unwired: 1 in]
                  n1335 = Not(x=w2083) -> (.not. x?=w2082:bool)
                }
              }
            }
            n1336 = Not(x=w2036) -> (.not. x?=w2035:bool)
            n1337 = case shown="True" w2035 {
              tunnel: w2033 -> [_ w2099]
              tunnel: w2031 -> [_ w2098]
              tunnel: w2034 -> [_ w2097]
              tunnel: w2032 -> [_ w2096]
              frame False {
              }
              frame True {
                w2092 = FALSE ("Get Point")
                n1338 = local read "Scan lines (y)"() -> (w2101:u64)
                n1339 = local read "Actual MCL Inc (V)"() -> (w2093:dbl)
                n1340 = local read "Scan steps (MCL)"() -> (w2100:u64)
                n1341 = Divide "Y Pix/step"(x=w2096, y=w2101) -> (x/y=w2108:dbl)
                n1342 = Divide "Y V/pix"(x=w2093, y=w2108) -> (x/y=w2107:dbl)
                n1343 = Divide "Y half step offset"(x=w2093, y=2.0) -> (x/y=w2109:dbl)
                n1344 = Divide "X pix/step"(x=w2097, y=w2100) -> (x/y=w2106:dbl)
                n1345 = Negate(x=w2109) -> (-x=w2110:dbl)
                n1346 = local read "Initial Y"() -> (w2116:dbl)
                n1347 = Multiply(x=w2098, y=w2107) -> (x*y=w2117:dbl)
                n1348 = Divide "X half step offset"(x=w2093, y=2.0) -> (x/y=w2103:dbl)
                n1349 = Divide "X V/pix"(x=w2093, y=w2106) -> (x/y=w2105:dbl)
                n1350 = Multiply(x=w2093, y=w2100) -> (x*y=w2112:dbl)
                n1351 = Compound Arithmetic op=ADD(w2110, w2117, w2116) -> (w2094:dbl)
                "Pointer Y (V)" <- w2094
                n1352 = Multiply(x=w2105, y=w2099) -> (x*y=w2114:dbl)
                n1353 = Negate(x=w2103) -> (-x=w2102:dbl)
                n1354 = local read "Initial X"() -> (w2115:dbl)
                n1355 = Negate(x=w2114) -> (-x=w2113:dbl)
                n1356 = Compound Arithmetic op=ADD(w2102, w2112, w2115, w2113) -> (w2095:dbl)
                "Pointer X (V)" <- w2095
                n1357 = Or(x="Set X Only", y="Set Confocal Spot (X-Y)") -> (x .or. y?=w2088:bool)
                n1358 = Or(x="Set Confocal Spot (X-Y)", y="Set Y Only") -> (x .or. y?=w2087:bool)
                n1359 = case shown="True" w2088 {
                  tunnel: w2095 -> [_ w2118]
                  frame False {
                  }
                  frame True {
                    n1360 = property on="AO2" class="Slide (strict)"("Val(Sgnl)"=w2118) -> ()  [unwired: 2 in, 2 out]
                  }
                }
                n1361 = case shown="True" w2087 {
                  tunnel: w2094 -> [_ w2119]
                  frame False {
                  }
                  frame True {
                    n1362 = property on="AO1" class="Slide (strict)"("Val(Sgnl)"=w2119) -> ()  [unwired: 2 in, 2 out]
                  }
                }
                n1363 = local write "Set Confocal Spot (X-Y)"(w2092) -> ()
                n1364 = local write "Set X Only"(w2092) -> ()
                n1365 = local write "Set Y Only"(w2092) -> ()
              }
            }
          }
          frame 3 {
            n1366 = local read "BD 2 Frequency 1 (MHz)"() -> (w2120:dbl)
            n1367 = local read "BD 1 Frequency 1 (MHz)"() -> (w2121:dbl)
            n1368 = local write "Manipulating Trap"(TRUE ("Manipulating Trap")) -> ()
            n1369 = local write "Coords"(T8 {"Horizontal"=0, "Vertical"=0} ("Coords")) -> ()
            n1370 = while {
              tunnel: w2126 -> [w2131]
